vi "PH_Cont-601k_PowerUnit.scr Stand by.vi"(0 "VI in":refnum<vi>, 5 "error in (no error)":errorcluster) -> (14 "VI out":refnum<vi>, 19 "error out":errorcluster)   [LabVIEW 2014, in "PH_Cont-601k_PowerUnit.lvlib"]
uses:
  PH_Cont-601k_PowerUnit.lvlib
  PH_Basics/PH_PowerUnit_BaseClass/PH_PowerUnit_BaseClass.SM States.ctl
  PH_Devices/PH_Cont-601k_PSU/PH_Cont-601k_PSU.Readyness.ctl
  PH_Devices/PH_Cont-601k_PSU/PH_Cont-601k_PSU.Readyness Program.ctl
  PH_Devices/PH_Cont-601k_PSU/PH_Cont-601k_PSU.Readyness Device.ctl
  PH_Basics/PH_PowerUnit_BaseClass/PH_PowerUnit_BaseClass.lvlib
  PH_Devices/PH_Cont-601k_PSU/PH_Cont-601k_PSU.lvlib
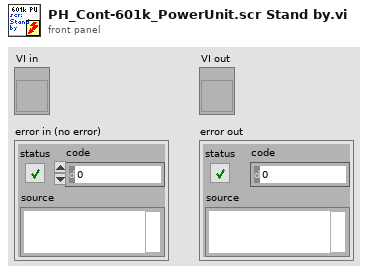
[diagram p1: front panel]
types:
  T1 = typedef "PH_Cont-601k_PSU.lvlib/PH_Cont-601k_PSU.Readyness.ctl" = cluster{"Program":T2, "Device":T3}
  T2 = typedef "PH_Cont-601k_PSU.lvlib/PH_Cont-601k_PSU.Readyness Program.ctl" = enum32{"OFF", "POWER", "INTERLOCK"}
  T3 = typedef "PH_Cont-601k_PSU.lvlib/PH_Cont-601k_PSU.Readyness Device.ctl" = enum32{"OFF", "CONNECTING", "CONNECTED", "OPERATING", "EOC", "ERROR"}
  T4 = typedef "PH_PowerUnit_BaseClass.lvlib/PH_PowerUnit_BaseClass.SM States.ctl" = enum16{".", "Stand by", "Switch PU on", "Configure", "Set Default Voltage", "Set STANDBY", "Set READY", "Wait for Shot Cmd", "Open Dump Rods", "Open Ross Relais", "Close Ross Relais", "Switch PSU on", "Switch PSU off", "Charge", "Switch GD Channel on", "Close Dump Rods", "Rods-TO", "RR-TO", "PSU-TO", "Trigger-TO"}
  T5 = typedef "PH_Cont-601k_PSU.lvlib/PH_Cont-601k_PSU.i attribute.ctl" = cluster{"GUI Refs":T6, "Interlock":bool, "Service ID applied Voltage":i32, "Device Settings":cluster{"Configuration":T7, "Flash Interval [s]":dbl, "Mode":T8, "Voltage [V]":u16, "Charge":bool, "VISA resource name":refnum<visa-resource-name>}, "Readyness":T1, "Information":cluster{"VISA resource name":refnum<visa-resource-name>, "Tagname Power On":string, "Interlock":cluster{"Instance":string, "Tagname":string}, "Limits [V]":cluster{"Lower":dbl, "Upper":dbl}, "Tagname PSU On":string}, "R2S":bool, "Charge is allowed":bool}
  T6 = typedef "PH_Cont-601k_PSU.lvlib/PH_Cont-601k_PSU.GUI Refs.ctl" = cluster{"Power On":refnum<vi>, "Hard- and Software":refnum<vi>, "Device Status":refnum<vi>, "Device Error":refnum<vi>, "Configuration":refnum<vi>, "Flash Interval [s]":refnum<vi>, "Interlock":refnum<vi>, "Interlock Indicator":refnum<vi>, "Voltage [V]":refnum<vi>, "Readyness":refnum<vi>, "Mode":refnum<vi>, "Reset Error":refnum<vi>, "Expert working":refnum<vi>, "Charge":refnum<vi>, "PSU On":refnum<vi>}
  T7 = typedef "PH_Cont-601k_PSU.lvlib/PH_Cont-601k_PSU.Configuration.ctl" = u16
  T8 = typedef "PH_Cont-601k_PSU.lvlib/PH_Cont-601k_PSU.Mode.ctl" = enum32{"STOP", "STANDBY", "READY", "EMISSION", "ERROR"}
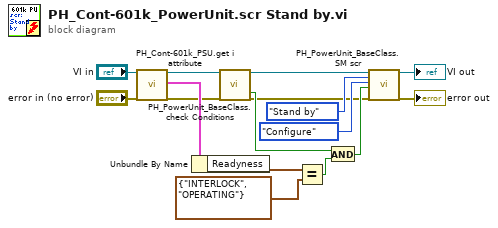
[diagram p0: block diagram]
diagram:
  n1 = call "PH_Cont-601k_PSU.get i attribute.vi"("i ref in"="VI in", "error in (no error)"="error in (no error)") -> ("i ref out"=w12:refnum<vi>, "i attribute"=w14:T5, "error out"=w11:errorcluster)  [unwired: 15 in]
  n2 = Unbundle By Name(w14) -> ("Readyness"=w15:T1)
  n3 = call "PH_PowerUnit_BaseClass.check Conditions.vi"("VI in"=w12, "error in (no error)"=w11) -> ("VI out"=w3:refnum<vi>, "Ready to switch PU on"=w16:bool, "error out"=w2:errorcluster)  [unwired: 14 in, 1 out]
  n4 = Equal?(x=w15, y=T1 {"Program"=enum."INTERLOCK", "Device"=enum."OPERATING"} ("Readyness")) -> (x = y?=w13:bool)
  n5 = And(x=w16, y=w13) -> (x .and. y?=w6:bool)
  n6 = call "PH_PowerUnit_BaseClass.SM scr.vi"("VI in"=w3, "Current SM State (condition)"=PH_PowerUnit_BaseClass.SM_States."Stand by", "Wanted SM State"=PH_PowerUnit_BaseClass.SM_States."Configure", "Further change condition"=w6, "error in (no error)"=w2) -> ("VI out"=→"VI out":refnum<vi>, "error out"=→"error out":errorcluster)  [unwired: 13 in]
